vi "Test Deserialize Variants.vi"(8 "error in (no error)":errorcluster) -> (0 "error out":errorcluster)   [LabVIEW 2017]
uses:
  src/Deserializer/JSON Deserializer/JSON Deserializer.lvclass
  <userlib>/_OpenG.lib/lvdata/lvdata.llb/Array of VData to VCluster__ogtk.vi
  <vilib>/addons/_JKI Toolkits/Caraya/classes/Test/Test.lvclass
  <vilib>/addons/_JKI Toolkits/Caraya/classes/Assert/Assert.lvclass
  src/JKI JSON Serialization.lvlib
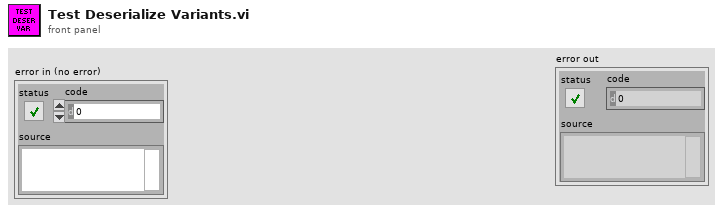
[diagram p1: front panel]
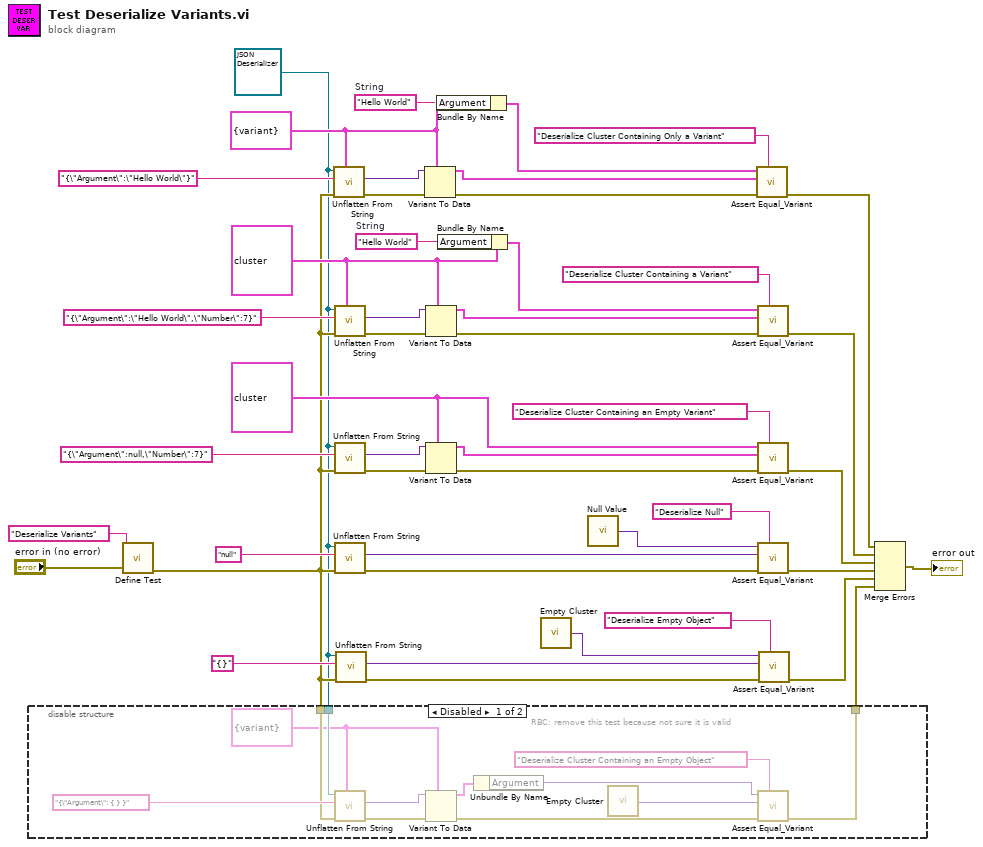
[diagram p0: block diagram]
diagram:
  w11 = cluster{"Argument":variant, "Number":i32} {"Argument"=variant, "Number"=7}
  w22 = "Hello World"  # String
  w25 = cluster{"Argument":variant} {"Argument"=variant}
  w35 = "Hello World"  # String
  w32 = cluster{"Argument":variant, "Number":i32} {"Argument"=variant, "Number"=7}
  w4 = refnum<class "JSON Deserializer.lvclass"> refnum ("Deserializer out")
  n1 = call <vilib>:"Define Test.vi"("error in (no error)"="error in (no error)", "Label (VI Title)"="Deserialize Variants") -> ("error out"=w5:errorcluster)  [unwired: 9 in]
  n2 = disable-structure shown="Disabled" {
    disable-tunnel: w5 -> [w53 _]
    disable-tunnel: w4 -> [w52 _]
    disable-tunnel: [w51 _] -> w3
    frame Disabled {
      w47 = cluster{"Argument":variant} {"Argument"=variant}
      # "RBC: remove this test because not sure it is valid"
      n3 = call-dynamic "Unflatten From String.vi"("Type and Defaults"=w47, "error in (no error)"=w53, "String"="{\"Argument\": { } }", "Deserializer in"=w52) -> ("error out"=w57:errorcluster, "Variant"=w56:variant)  [unwired: 5 in, 1 out]
      n4 = Variant To Data(error in=w57, type=w47, Variant=w56) -> (data=w50:cluster{"Argument":variant}, error out=w58:errorcluster)
      n5 = Unbundle By Name(w50) -> ("Argument"=w49:variant)
      n6 = call "Empty Cluster.vi"() -> ("Empty Cluster"=w48:variant)
      n7 = call <vilib>:"Assert Equal_Variant.vi"("Label"="Deserialize Cluster Containing an Empty Object", "error in (no error)"=w58, "Y"=w48, "X"=w49) -> ("error out"=w51:errorcluster)  [unwired: 7 in]
    }
    frame Enabled {
    }
  }
  n8 = call-dynamic "Unflatten From String.vi"("Type and Defaults"=w25, "error in (no error)"=w5, "String"="{\"Argument\":\"Hello World\"}", "Deserializer in"=w4) -> ("error out"=w24:errorcluster, "Variant"=w23:variant)  [unwired: 5 in, 1 out]
  n9 = call-dynamic "Unflatten From String.vi"("Type and Defaults"=w32, "error in (no error)"=w5, "String"="{\"Argument\":\"Hello World\",\"Number\":7}", "Deserializer in"=w4) -> ("error out"=w33:errorcluster, "Variant"=w34:variant)  [unwired: 5 in, 1 out]
  n10 = call-dynamic "Unflatten From String.vi"("error in (no error)"=w5, "String"="{\"Argument\":null,\"Number\":7}", "Deserializer in"=w4) -> ("error out"=w16:errorcluster, "Variant"=w15:variant)  [unwired: 6 in, 1 out]
  n11 = call-dynamic "Unflatten From String.vi"("error in (no error)"=w5, "String"="null", "Deserializer in"=w4) -> ("error out"=w40:errorcluster, "Variant"=w39:variant)  [unwired: 6 in, 1 out]
  n12 = call-dynamic "Unflatten From String.vi"("error in (no error)"=w5, "String"="{}", "Deserializer in"=w4) -> ("error out"=w8:errorcluster, "Variant"=w7:variant)  [unwired: 6 in, 1 out]
  n13 = Variant To Data(error in=w24, type=w25, Variant=w23) -> (data=w26:cluster{"Argument":variant}, error out=w28:errorcluster)
  n14 = Variant To Data(error in=w33, type=w32, Variant=w34) -> (data=w31:cluster{"Argument":variant, "Number":i32}, error out=w29:errorcluster)
  n15 = Variant To Data(error in=w16, type=w11, Variant=w15) -> (data=w17:cluster{"Argument":variant, "Number":i32}, error out=w18:errorcluster)
  n16 = Bundle By Name(cluster=w25, "Argument"=w22) -> (w27:cluster{"Argument":variant})
  n17 = Bundle By Name(cluster=w32, "Argument"=w35) -> (w30:cluster{"Argument":variant, "Number":i32})
  n18 = call "Empty Cluster.vi"() -> ("Empty Cluster"=w1:variant)
  n19 = call "Null Value.vi"() -> ("Null"=w2:variant)
  n20 = call <vilib>:"Assert Equal_Variant.vi"("Label"="Deserialize Cluster Containing Only a Variant", "error in (no error)"=w28, "Y"=w26, "X"=w27) -> ("error out"=w19:errorcluster)  [unwired: 7 in]
  n21 = call <vilib>:"Assert Equal_Variant.vi"("Label"="Deserialize Cluster Containing a Variant", "error in (no error)"=w29, "Y"=w31, "X"=w30) -> ("error out"=w37:errorcluster)  [unwired: 7 in]
  n22 = call <vilib>:"Assert Equal_Variant.vi"("Label"="Deserialize Cluster Containing an Empty Variant", "error in (no error)"=w18, "Y"=w17, "X"=w11) -> ("error out"=w12:errorcluster)  [unwired: 7 in]
  n23 = call <vilib>:"Assert Equal_Variant.vi"("Label"="Deserialize Null", "error in (no error)"=w40, "Y"=w39, "X"=w2) -> ("error out"=w43:errorcluster)  [unwired: 7 in]
  n24 = call <vilib>:"Assert Equal_Variant.vi"("Label"="Deserialize Empty Object", "error in (no error)"=w8, "Y"=w7, "X"=w1) -> ("error out"=w6:errorcluster)  [unwired: 7 in]
  n25 = Merge Errors(w19, w37, w12, w43, w6, w3) -> (→"error out":errorcluster)
